vi "Assert Collection Empty.vi"(7 "Message (\"\")":string, 8 "error in (no error)":errorcluster, 10 "Collection":variant) -> (0 "error out":errorcluster)   [LabVIEW 2017, in "Transparent Assertions.lvlib"]
doc: "Asserts that a collection (array, set, or map) is empty. Returns an error if the assertion fails, and optionally appends a custom message to the error."
uses:
  Transparent Assertions.lvlib
  Collection Is Empty/Collection Is Empty.lvclass
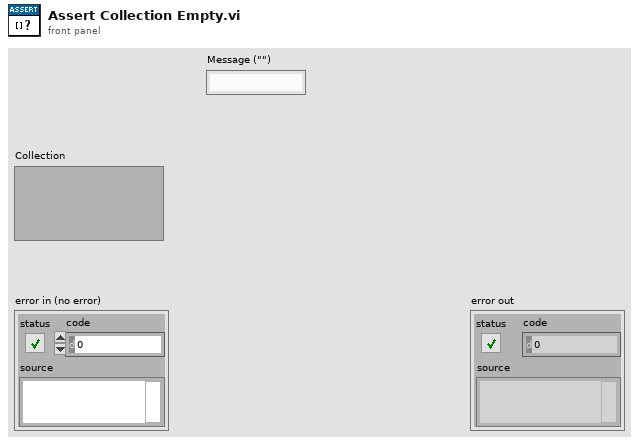
[diagram p1: front panel]
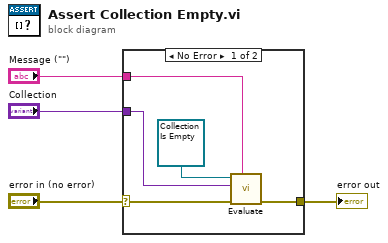
[diagram p0: block diagram]
diagram:
  n1 = case shown="No Error" "error in (no error)" {
    selector: "error in (no error)" -> [w5 w10]
    tunnel: [w9 w10] -> w4
    tunnel: "Collection" -> [w8 _]
    tunnel: "Message (\"\")" -> [w7 _]
    frame No Error {
      n2 = call-dynamic "Evaluate.vi"("Message (\"\")"=w7, "error in (no error)"=w5, "Actual"=w8, "Constraint in"=refnum<class "Collection Is Empty.lvclass"> refnum ("Transparent Assertions.lvlib:Constraints.lvlib:Collection Is Empty.lvclass")) -> ("error out"=w9:errorcluster)  [unwired: 6 in, 1 out]
    }
    frame Error {
    }
  }
  "error out" <- w4
